vi "Set Wheel Width.vi"(8 "error in (no error)":errorcluster, 10 "Width (m)":dbl, 11 "Rover in":refnum<class "Rover.lvclass">) -> (0 "error out":errorcluster, 3 "Rover out":refnum<class "Rover.lvclass">)   [LabVIEW 2020]
uses:
  Rover.lvclass
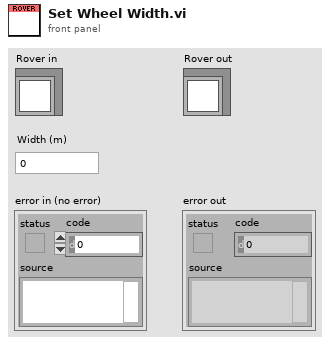
[diagram p1: front panel]
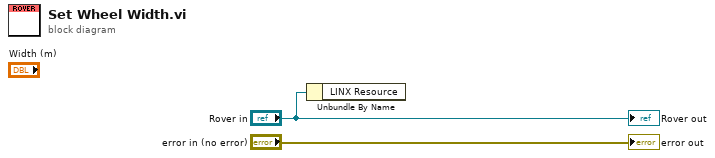
[diagram p0: block diagram]
diagram:
  n1 = Unbundle By Name("Rover in") -> ()  [unwired: 1 out]
  "error out" <- "error in (no error)"
  "Rover out" <- "Rover in"
